vi "Write Interactive.vi"(8 "error in (no error)":errorcluster, 10 "Interactive":bool, 11 "DefineSuite in":refnum<class "DefineSuite.lvclass">) -> (0 "error out":errorcluster, 3 "DefineSuite out":refnum<class "DefineSuite.lvclass">)   [LabVIEW 2021, in "Bananas.lvlib" / "DefineSuite.lvclass"]
uses:
  DefineSuite.lvclass
  DefineSuite.lvclass/DefineSuite.ctl
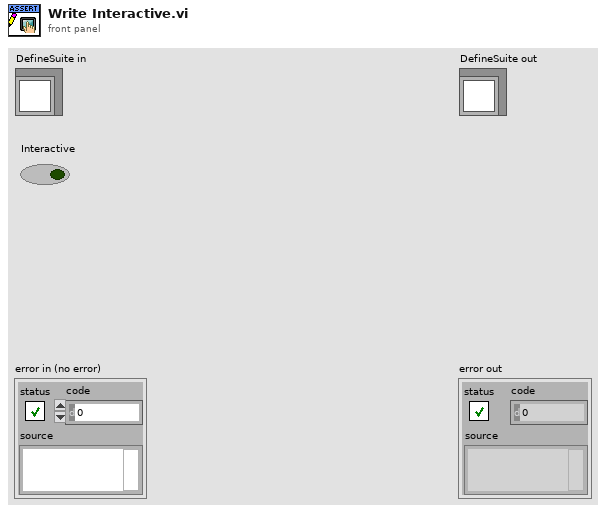
[diagram p1: front panel]
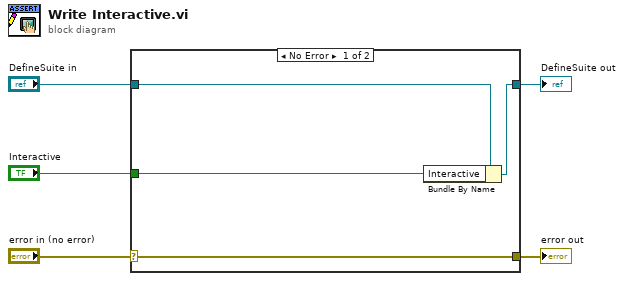
[diagram p0: block diagram]
diagram:
  n1 = case shown="No Error" "error in (no error)" {
    selector: "error in (no error)" -> [w9 w10]
    tunnel: [w9 w10] -> w4
    tunnel: [w7 w11] -> w2
    tunnel: "DefineSuite in" -> [w8 w11]
    tunnel: "Interactive" -> [w6 _]
    frame No Error {
      n2 = Bundle By Name(cluster=w8, "Interactive"=w6) -> (w7:refnum<class "DefineSuite.lvclass">)
    }
    frame Error {
    }
  }
  "error out" <- w4
  "DefineSuite out" <- w2
